vi "Matrix Power.vi"   [LabVIEW 2017, in "NI_AALBase.lvlib"]
doc: "Computes the nth power of <B>Input Matrix</B>. Wire data to the <B>Input Matrix</B> input to determine the polymorphic instance to use or manually select the instance."
uses:
  NI_AALBase.lvlib
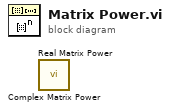
[diagram p0: block diagram]
diagram:
  n1 = call "Complex Matrix Power.vi"() -> ()  [unwired: 2 in, 2 out]
  n2 = call "Real Matrix Power.vi"() -> ()  [unwired: 2 in, 2 out]
